vi "initialization.vi"(8 "error in (no error)":errorcluster, 11 "DAQmxTaskContainer in":refnum<class "DAQmxTaskContainer.lvclass">) -> (0 "error out":errorcluster, 3 "DAQmxTaskContainer out":refnum<class "DAQmxTaskContainer.lvclass">)   [LabVIEW 2015, in "DAQmxTaskContainer.lvclass"]
uses:
  DAQmxTaskContainer.lvclass
  GeneralFunctionality/GeneralFunctionality.lvclass/GeneralFunctionality.ctl
  Config/Config.lvclass/Config.ctl
  dependecies/ControlsVIs/Clusters-def/list-of-keys-DAQmx-tasks.ctl
  DAQmxTasklDInput/DAQmxTaskDInput.lvclass
  DAQmxTaskAICurrent.lvclass
  DAQmxTaskAICurrent_General/DAQmxTaskAICurrent_General.lvclass/DAQmxTaskAICurrent_General.ctl
  DAQmxTaskAITension/DAQmxTaskAIVoltage.lvclass
  DAQmxTaskAITension_General/DAQmxTaskAIVoltage_General.lvclass/DAQmxTaskAIVoltage_General.ctl
  DAQmxTaskDOutput/DAQmxTaskDOutput.lvclass
  DAQmxTaksCounterDigital/DAQmxTaskCounterDigital.lvclass
  DAQmxTaskContainer_General/DAQmxTaksContainer_General.lvclass/DAQmxTaksContainer_General.ctl
  Config/Config.lvclass
  DAQmxTask.lvclass
  DAQmxTaskContainer_General/DAQmxTaksContainer_General.lvclass
  GeneralFunctionality/GeneralFunctionality.lvclass
  DAQmxTaskAICurrent_General/DAQmxTaskAICurrent_General.lvclass
  DAQmxTaskAITension_General/DAQmxTaskAIVoltage_General.lvclass
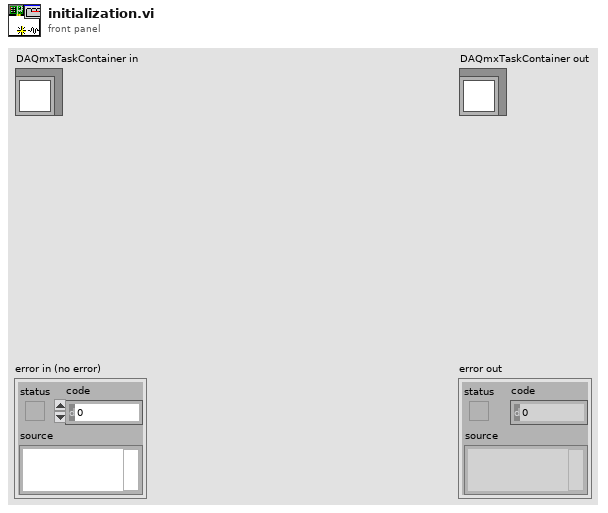
[diagram p1: front panel]
types:
  T1 = typedef "DAQmxTaksContainer_General.lvclass/list-of-keys-DAQmx-tasks.ctl" = string
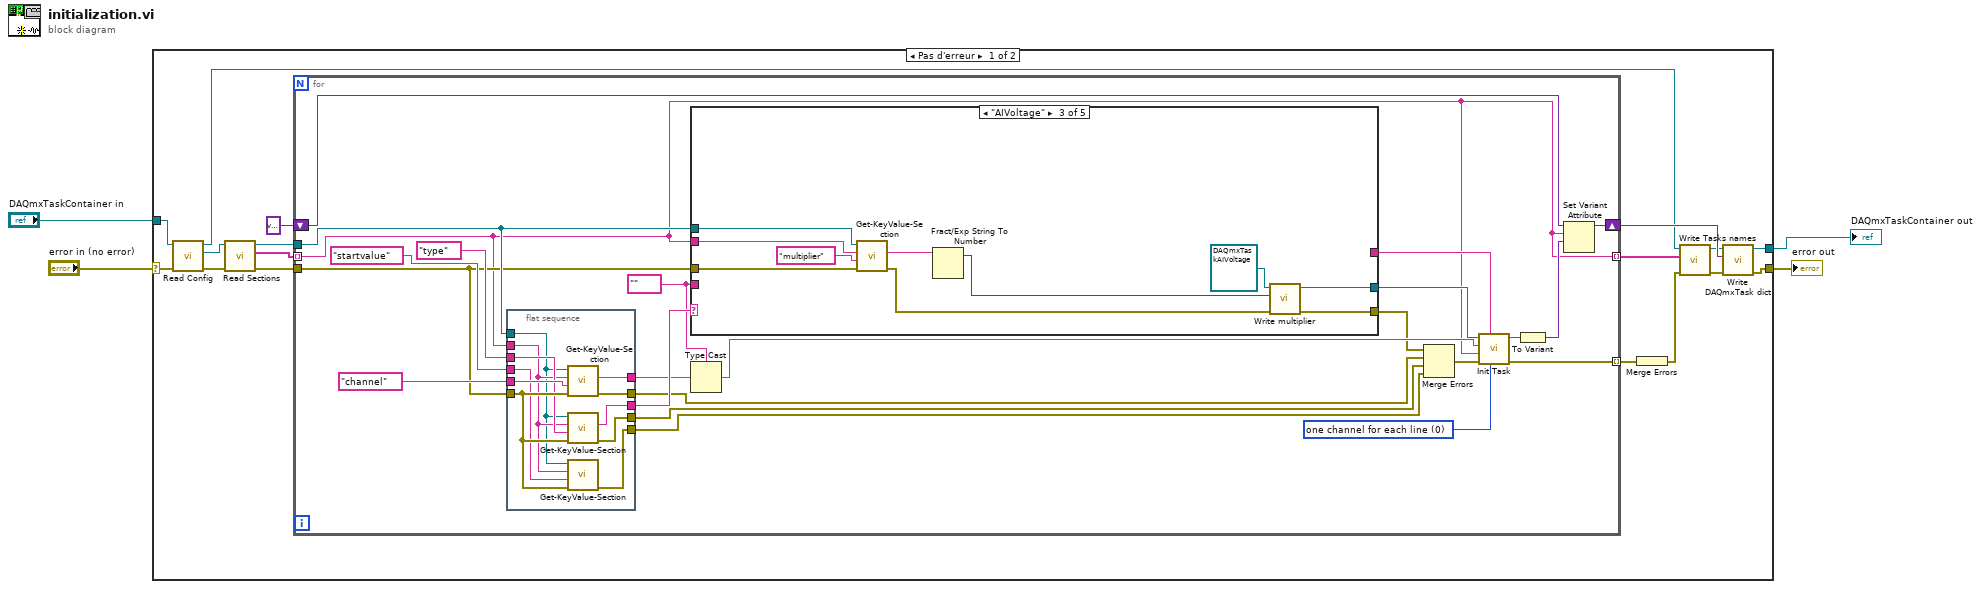
[diagram p0: block diagram]
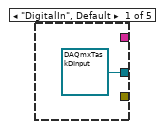
[diagram p2: hidden frame]
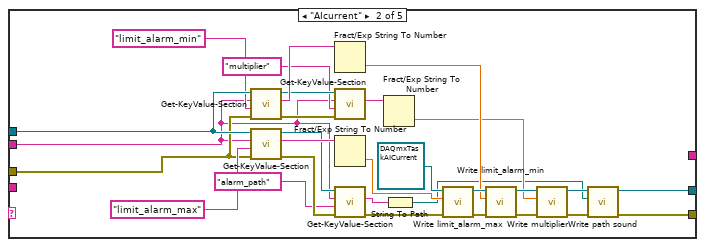
[diagram p3: hidden frame]
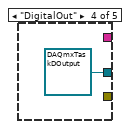
[diagram p4: hidden frame]
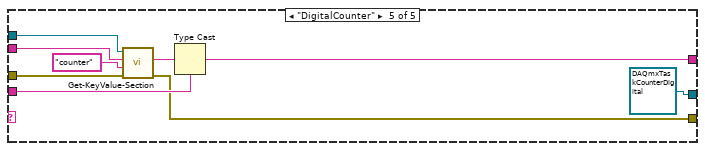
[diagram p5: hidden frame]
diagram:
  n1 = case shown="Pas d'erreur" "error in (no error)" {
    selector: "error in (no error)" -> [w8 w107]
    tunnel: [w11 w107] -> w3
    tunnel: [w10 w106] -> w1
    tunnel: "DAQmxTaskContainer in" -> [w9 w106]
    frame No Error {
      n2 = call "Read Config.vi"("error in (no error)"=w8, "GeneralFunctionality en entrée"=w9) -> ("error out"=w7:errorcluster, "Config.lvclass"=w6:refnum<class "Config.lvclass">, "GeneralFunctionality en sortie"=w5:refnum<class "DAQmxTaskContainer.lvclass">)  [unwired: 7 in]
      n3 = call "Read Sections.vi"("error in (no error)"=w7, "Config in"=w6) -> ("error out"=w14:errorcluster, "Sections"=w13:string[], "Config out"=w19:refnum<class "Config.lvclass">)  [unwired: 7 in]
      n4 = for {
        tunnel: w13 -> [w22] mode=indexing
        tunnel: w14 -> [w24]
        tunnel: w19 -> [w39]
        shift-right: [w30] -> w18
        shift-left: variant -> [w31]
        tunnel: [w29] -> w12 mode=indexing
        tunnel: [w22] -> w16 mode=indexing
        w34 = 0 items=["one channel for each line", "one channel for all lines"] ("line grouping")
        w26 = tag "" ("physical channels")
        n5 = flat-sequence {
          tunnel: w24 -> [w55]
          tunnel: T1 "channel" ("Key") -> [w54]
          tunnel: T1 "type" ("Key") -> [w53]
          tunnel: T1 "startvalue" ("Key") -> [w52]
          tunnel: [w51] -> w41
          tunnel: [w50] -> w40
          tunnel: w22 -> [w49]
          tunnel: w39 -> [w48]
          tunnel: [w47] -> w38
          tunnel: [w46] -> w37
          tunnel: [w45] -> w36
          frame #0 {
            n6 = call-dynamic "Get-KeyValue-Section.vi"("error in (no error)"=w55, "Key"=w54, "Section"=w49, "Config in"=w48) -> ("error out"=w47:errorcluster, "Value"=w50:string)  [unwired: 5 in, 1 out]
            n7 = call-dynamic "Get-KeyValue-Section.vi"("error in (no error)"=w55, "Key"=w53, "Section"=w49, "Config in"=w48) -> ("error out"=w46:errorcluster, "Value"=w51:string)  [unwired: 5 in, 1 out]
            n8 = call-dynamic "Get-KeyValue-Section.vi"("error in (no error)"=w55, "Key"=w52, "Section"=w49, "Config in"=w48) -> ("error out"=w45:errorcluster)  [unwired: 5 in, 2 out]
          }
        }
        n9 = case shown="\"AIVoltage\"" w41 {
          tunnel: w39 -> [_ w73 w92 _ w100]
          tunnel: [refnum<class "DAQmxTaskDInput.lvclass"> refnum ("DAQmxTaskDInput.lvclass") w81 w86 refnum<class "DAQmxTaskDOutput.lvclass"> refnum ("DAQmxTaskDOutput.lvclass") refnum<class "DAQmxTaskCounterDigital.lvclass"> refnum ("DAQmxTaskCounterDigital.lvclass")] -> w33
          tunnel: w26 -> [_ _ _ _ w104]
          tunnel: [_ _ _ _ w102] -> w25
          tunnel: w22 -> [_ w60 w93 _ w101]
          tunnel: w24 -> [_ w68 w91 _ w98]
          tunnel: [_ w77 w87 _ w97] -> w23
          frame "DigitalIn", Default {
          }
          frame "AIcurrent" {
            n10 = call-dynamic "Get-KeyValue-Section.vi"("error in (no error)"=w68, "Key"="limit_alarm_min", "Section"=w60, "Config in"=w73) -> ("error out"=w67:errorcluster, "Value"=w71:string, "Config out"=w69:refnum<class "Config.lvclass">)  [unwired: 5 in]
            n11 = call-dynamic "Get-KeyValue-Section.vi"("error in (no error)"=w68, "Key"="limit_alarm_max", "Section"=w60, "Config in"=w73) -> ("error out"=w63:errorcluster, "Value"=w75:string, "Config out"=w61:refnum<class "Config.lvclass">)  [unwired: 5 in]
            n12 = Fract/Exp String To Number(string=w71) -> (number=w70:dbl)  [unwired: 3 in, 1 out]
            n13 = call-dynamic "Get-KeyValue-Section.vi"("error in (no error)"=w67, "Key"="multiplier", "Section"=w60, "Config in"=w69) -> ("Value"=w65:string)  [unwired: 5 in, 2 out]
            n14 = Fract/Exp String To Number(string=w75) -> (number=w74:dbl)  [unwired: 3 in, 1 out]
            n15 = call-dynamic "Get-KeyValue-Section.vi"("error in (no error)"=w63, "Key"="alarm_path", "Section"=w60, "Config in"=w61) -> ("error out"=w62:errorcluster, "Value"=w58:string)  [unwired: 5 in, 1 out]
            n16 = Fract/Exp String To Number(string=w65) -> (number=w64:dbl)  [unwired: 3 in, 1 out]
            n17 = String To Path(string=w58) -> (path=w57:path)
            n18 = call "Write limit_alarm_max.vi"("error in (no error)"=w62, "limit_alarm_max"=w74, "DAQmxTaskAICurrent_General in"=refnum<class "DAQmxTaskAICurrent.lvclass"> refnum ("DAQmxTaskAICurrent.lvclass")) -> ("error out"=w80:errorcluster, "DAQmxTaskAICurrent_General out"=w84:refnum<class "DAQmxTaskAICurrent.lvclass">)  [unwired: 7 in]
            n19 = call "Write limit_alarm_min.vi"("error in (no error)"=w80, "limit_alarm_min"=w70, "DAQmxTaskAICurrent_General in"=w84) -> ("error out"=w79:errorcluster, "DAQmxTaskAICurrent_General out"=w83:refnum<class "DAQmxTaskAICurrent.lvclass">)  [unwired: 7 in]
            n20 = call "Write multiplier.vi"("error in (no error)"=w79, "multiplier"=w64, "DAQmxTaskAICurrent_General in"=w83) -> ("error out"=w78:errorcluster, "DAQmxTaskAICurrent_General out"=w82:refnum<class "DAQmxTaskAICurrent.lvclass">)  [unwired: 7 in]
            n21 = call "Write path sound.vi"("error in (no error)"=w78, "path sound"=w57, "DAQmxTaskAICurrent_General in"=w82) -> ("error out"=w77:errorcluster, "DAQmxTaskAICurrent_General out"=w81:refnum<class "DAQmxTaskAICurrent.lvclass">)  [unwired: 7 in]
          }
          frame "AIVoltage" {
            n22 = call-dynamic "Get-KeyValue-Section.vi"("error in (no error)"=w91, "Key"="multiplier", "Section"=w93, "Config in"=w92) -> ("error out"=w89:errorcluster, "Value"=w94:string)  [unwired: 5 in, 1 out]
            n23 = Fract/Exp String To Number(string=w94) -> (offset past number=w88:i32)  [unwired: 3 in, 1 out]
            n24 = call "Write multiplier.vi"("error in (no error)"=w89, "multiplier"=w88, "DAQmxTaskAIVoltage_General in"=refnum<class "DAQmxTaskAIVoltage.lvclass"> refnum ("DAQmxTaskAIVoltage.lvclass")) -> ("error out"=w87:errorcluster, "DAQmxTaskAIVoltage_General out"=w86:refnum<class "DAQmxTaskAIVoltage.lvclass">)  [unwired: 7 in]
          }
          frame "DigitalOut" {
          }
          frame "DigitalCounter" {
            n25 = call-dynamic "Get-KeyValue-Section.vi"("error in (no error)"=w98, "Key"="counter", "Section"=w101, "Config in"=w100) -> ("error out"=w97:errorcluster, "Value"=w103:string)  [unwired: 5 in, 1 out]
            n26 = Type Cast(type=w104, x=w103) -> (*(type *) &x=w102:tag)
          }
        }
        n27 = Type Cast(type=w26, x=w40) -> (*(type *) &x=w35:tag)
        n28 = Merge Errors(w23, w38, w37, w36) -> (w32:errorcluster)
        n29 = call-dynamic "Init Task.vi"("line grouping"=w34, "counter"=w25, "error in (no error)"=w32, "name"=w22, "physical channels"=w35, "DAQmxTask in"=w33) -> ("error out"=w29:errorcluster, "DAQmxTask out"=w27:refnum<class "DAQmxTask.lvclass">)  [unwired: 4 in]
        n30 = To Variant(anything=w27) -> (Variant=w28:variant)
        n31 = Set Variant Attribute(Variant=w31, name=w22, value=w28) -> (Variant out=w30:variant)  [unwired: 1 in, 2 out]
      }
      n32 = Merge Errors(w12) -> (w21:errorcluster)
      n33 = call "Write Tasks names.vi"("error in (no error)"=w21, "Tasks names"=w16, "DAQmxTaskContainer_general en entrée"=w5) -> ("error out"=w20:errorcluster, "DAQmxTaskContainer_general en sortie"=w17:refnum<class "DAQmxTaskContainer.lvclass">)  [unwired: 7 in]
      n34 = call-dynamic "Write DAQmxTask dict.vi"("error in (no error)"=w20, "DAQmxTask dict"=w18, "DAQmxTaskContainer_general in"=w17) -> ("error out"=w11:errorcluster, "DAQmxTaskContainer_general out"=w10:refnum<class "DAQmxTaskContainer.lvclass">)  [unwired: 7 in]
    }
    frame Error {
    }
  }
  "error out" <- w3
  "DAQmxTaskContainer out" <- w1
